vi "FormatDateIntoUtcString.vi"(11 "Date (UTC)":timestamp format="%<%H:%M:%S%3u\n%Y/%m/%d>T") -> (3 "Formatted Date (UTC)":string)   [LabVIEW 2019, in "Asset.lvclass"]
uses:
  Asset/Asset.lvclass
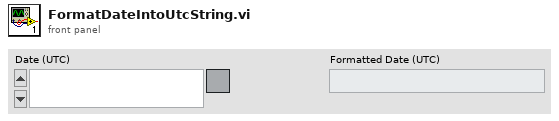
[diagram p1: front panel]
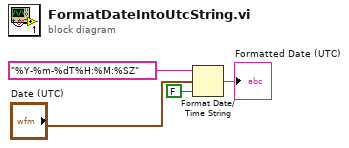
[diagram p0: block diagram]
diagram:
  n1 = Format Date/Time String(time format string (%c)="%Y-%m-%dT%H:%M:%SZ", seconds (now)="Date (UTC)", UTC format=FALSE) -> (date/time string=→"Formatted Date (UTC)":string)
